vi "DeppPutRegRepeat.vi"(7 "Overlap?":bool, 8 "Error In":errorcluster, 9 "Data":u8[](array[numeric]), 10 "Address":u8, 11 "Device Handle":u32) -> (0 "Error Out":errorcluster, 3 "Device Handle":u32)   [LabVIEW 2011, in "LVH-Adept.lvlib" / "DEPP.lvlib"]
uses:
  <vilib>/LabVIEW Hacker/Adept/Private/DEPP/DEPP.lvlib
  <vilib>/LabVIEW Hacker/Adept/Private/DEPP/Private/Type Defs/Error.ctl
  <vilib>/LabVIEW Hacker/Adept/Private/Resources/depp.dll
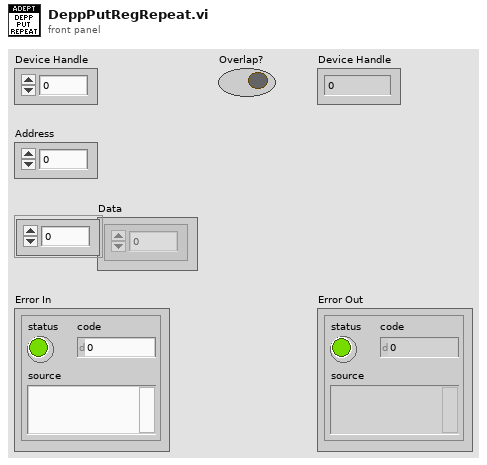
[diagram p1: front panel]
types:
  T1 = typedef "LVH-Adept.lvlib/DEPP.lvlib/Error.ctl" = enum16{"Unknown", "Enable", "Enable Port", "Get Register", "Get Register Repeat", "Get Register Set", "Put Register", "Put Register Repeat", "Put Register Set", "Disable", "Set Pair Size"}
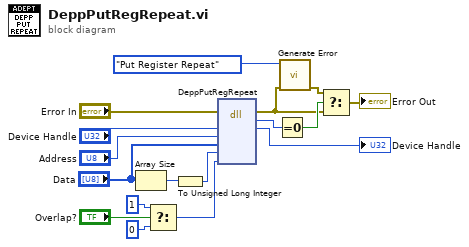
[diagram p0: block diagram]
diagram:
  n1 = Array Size(array="Data") -> (size(s)=w2:i32)
  n2 = Select(t=u8 1, s="Overlap?", f=u8 0) -> (s? t:f=w4:u8)
  n3 = To Unsigned Long Integer(number=w2) -> (unsigned 32bit integer=w1:u32)
  n4 = dll-call lib="C:/Program Files (x86)/National Instruments/LabVIEW 2011/vi.lib/LabVIEW Hacker/Adept/Private/Resources/depp.dll" fn="DeppPutRegRepeat"(error in="Error In", "hif"="Device Handle", "bAddr"="Address", "bData"="Data", "cbData"=w1, "fOverlap"=w4) -> (error out=w9:errorcluster, "Success"=w16:u32, "hif"=→"Device Handle":u32)  [unwired: 6 in, 1 out]
  n5 = Equal To 0?(x=w16) -> (x = 0?=w15:bool)
  n6 = call <vilib>:"Generate Error.vi"("Error In"=w9, "DEPP Error"=Error."Put Register Repeat") -> ("Error Out"=w10:errorcluster)  [unwired: 9 in]
  n7 = Select(t=w10, s=w15, f=w9) -> (s? t:f=→"Error Out":errorcluster)
